vi "T to XYZOAT.vi"(9 "T":T2 format="%.3f") -> (1 "XYZOAT":T1)   [LabVIEW 2013]
uses:
  <vilib>/Analysis/Matrix/Datatypes/RealMatrix.ctl
  <vilib>/Analysis/Matrix/NI_Matrix.lvlib
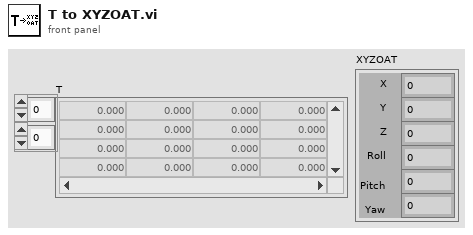
[diagram p1: front panel]
types:
  T1 = cluster{"X":dbl, "Y":dbl, "Z":dbl, "Roll":dbl, "Pitch":dbl, "Yaw":dbl}
  T2 = typedef "NI_Matrix.lvlib/RealMatrix.ctl" = dbl[][]
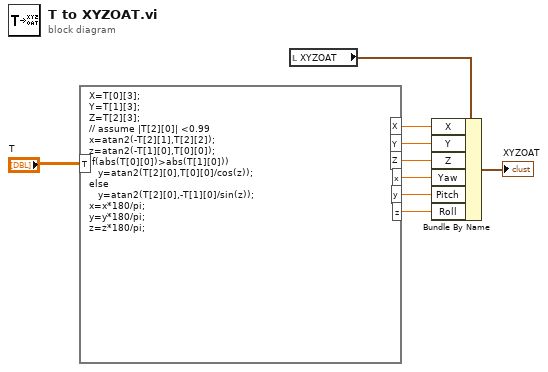
[diagram p0: block diagram]
diagram:
  n1 = formula code="X=T[0][3];\nY=T[1][3];\nZ=T[2][3];\n// assume |T[2][0]| <0.99\nx=atan2(-T[2][1],T[2][2]);\nz=atan2(-T[1][0],T[0][0]);\nif(abs(T[0][0])>abs(T[1][0]))\n   y=atan2(T[2][0],T[0][0]/cos(z));\nelse\n   y=atan2(T[2][0],-T[1][0]/sin(z));\nx=x*180/pi;\ny=y*180/pi;\nz=z*180/pi;"("T"="T") -> ("X"=w7:dbl, "Y"=w6:dbl, "Z"=w5:dbl, "x"=w3:dbl, "y"=w2:dbl, "z"=w1:dbl)
  n2 = local read "XYZOAT"() -> (w8:T1)
  n3 = Bundle By Name(cluster=w8, "X"=w7, "Y"=w6, "Z"=w5, "Yaw"=w3, "Pitch"=w2, "Roll"=w1) -> (→"XYZOAT":T1)
